vi "RMS (10 or 12 Cycles).vi"(0 "complex spectra":T2(array[cluster]), 9 "system info in":refnum<class "EP System Info.lvclass">, 11 "error in (no error)":errorcluster) -> (4 "RMS values":dbl[](array[numeric]), 10 "system info out":refnum<class "EP System Info.lvclass">, 15 "error out":errorcluster)   [LabVIEW 2014, in "NI_EP_Power Quality.lvlib"]
doc: "Calculates the RMS voltage value or RMS current value of a complex spectrum for a 10/12-cycle block, according to IEC 61000-4-30:2008.\n\nThis VI supports measuring single-line and multiple-line systems."
uses:
  <vilib>/addons/Electrical Power/PQ/NI_EP_Power Quality.lvlib
  <vilib>/addons/Electrical Power/PQ/Common/Controls/ep_AI Data Channel.ctl
  <vilib>/addons/Electrical Power/PQ/Common/Classes/System Info/EP System Info.lvclass
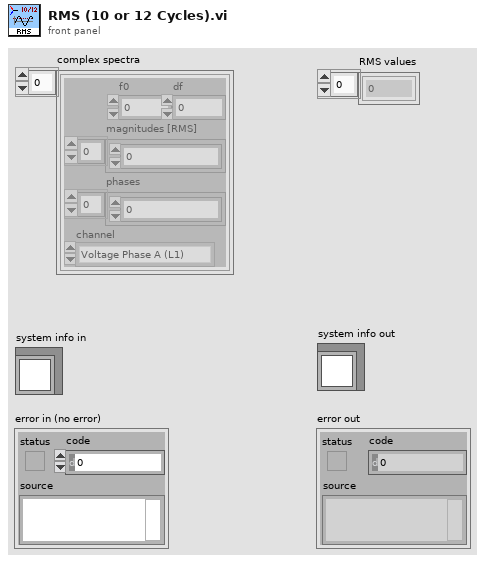
[diagram p1: front panel]
types:
  T1 = typedef "NI_EP_Power Quality.lvlib/ep_AI Data Channel.ctl" = enum16{"Voltage Phase A (L1)", "Voltage Phase B (L2)", "Voltage Phase C (L3)", "Voltage Phase N (Neutral)", "Current Phase A (L1)", "Current Phase B (L2)", "Current Phase C (L3)", "Current Phase N (Neutral)"}
  T2 = cluster{"f0":dbl, "df":dbl, "magnitudes [RMS]":dbl[], "phases":dbl[], "channel":T1}[]
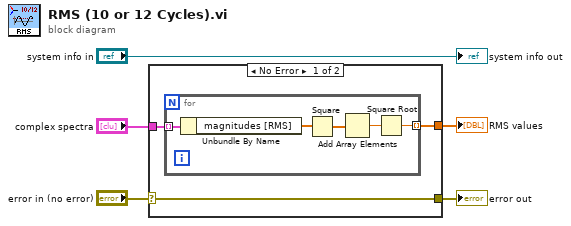
[diagram p0: block diagram]
diagram:
  n1 = case shown="No Error" "error in (no error)" {
    selector: "error in (no error)" -> [w6 w14]
    tunnel: "complex spectra" -> [w8 _]
    tunnel: [w7 _] -> w3
    tunnel: [w6 w14] -> w1
    frame No Error {
      n2 = for {
        tunnel: w8 -> [w13] mode=indexing
        tunnel: [w10] -> w7 mode=indexing
        n3 = Unbundle By Name(w13) -> ("magnitudes [RMS]"=w9:dbl[])
        n4 = Square(x=w9) -> (x^2=w12:dbl[])
        n5 = Add Array Elements(numeric array=w12) -> (sum=w11:dbl)
        n6 = Square Root(x=w11) -> (sqrt(x)=w10:dbl)
      }
    }
    frame Error {
    }
  }
  "error out" <- w1
  "RMS values" <- w3
  "system info out" <- "system info in"
